vi "Clean frame address.vi"(11 "Initial address counter in":u32) -> (3 "Initial address counter out":u32)   [LabVIEW 2015]
uses:
  OpenScan Labview code_20170126/Global_Sample per Frame.vi
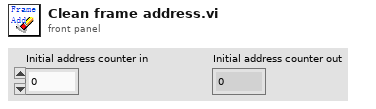
[diagram p1: front panel]
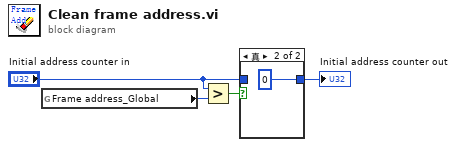
[diagram p0: block diagram]
diagram:
  n1 = global read "Global_Sample per Frame.vi" "Frame address_Global"() -> (w1:u32)
  n2 = Greater?(x="Initial address counter in", y=w1) -> (0:w2:bool)
  n3 = case shown="真" w2 {
    tunnel: [w5 u32 0 ("Initial address counter")] -> w3
    tunnel: "Initial address counter in" -> [w5 _]
    frame False {
    }
    frame True {
    }
  }
  "Initial address counter out" <- w3
